vi "SendIntegrationControl.vi"(8 "error in (no error)":errorcluster, 10 "Integration Control Register":T1 items=["UNDEFINED"=0, "NAVX_INTEGRATION_CTL_RESET_VEL_X"=1, "NAVX_INTEGRATION_CTL_RESET_VEL_Y"=2, "NAVX_INTEGRATION_CTL_RESET_VEL_Z"=4, "NAVX_INTEGRATION_CTL_RESET_DISP_X"=8, "NAVX_INTEGRATION_CTL_RESET_DISP_Y"=16, "NAVX_INTEGRATION_CTL_RESET_DISP_Z"=32, "NAVX_INTEGRATION_CTL_RESET_YAW"=128], 11 "navX - I2C in":refnum<class "navX - I2C.lvclass">) -> (0 "error out":errorcluster, 3 "navX - I2C out":refnum<class "navX - I2C.lvclass">)   [LabVIEW 2015, in "navX Library v3.lvlib" / "navX - I2C.lvclass"]
uses:
  navX - I2C.lvclass
  navX - Interface/_TypeDefs/IntegrationControlRegisterTypeDef.ctl
  navX Registry Cache/_TypeDefs/DeviceRegistryTypeDef.ctl
  navX - I2C.lvclass/navX - I2C.ctl
  navX - Interface/navX - Interface.lvclass
  navX Registry Cache/navX Registry Cache.lvclass
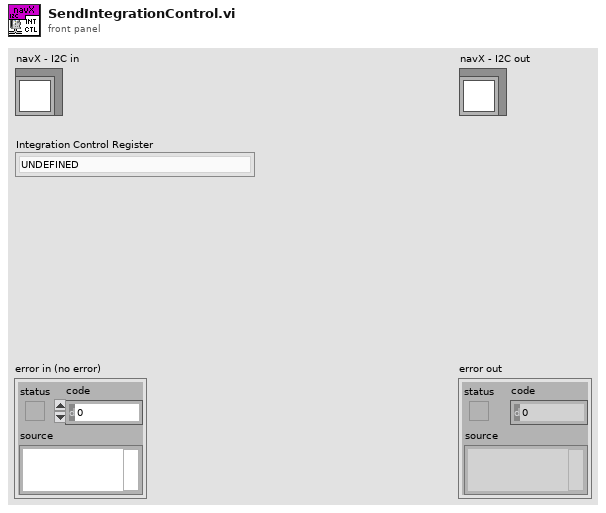
[diagram p1: front panel]
types:
  T1 = typedef "navX Library v3.lvlib/navX - Interface.lvclass/IntegrationControlRegisterTypeDef.ctl" = u8
  T2 = typedef "navX Library v3.lvlib/navX Registry Cache.lvclass/DeviceRegistryTypeDef.ctl" = u8
  T3 = typedef "WPI_I2CDevRef.ctl" = cluster{"DevStatus":errorcluster, "Device Address":u8, "Handle":i32, "I2C Bus":T4}
  T4 = typedef "i2c_bus.ctl" = enum16{"I2C On-Board", "I2C MXP", "Invalid"}
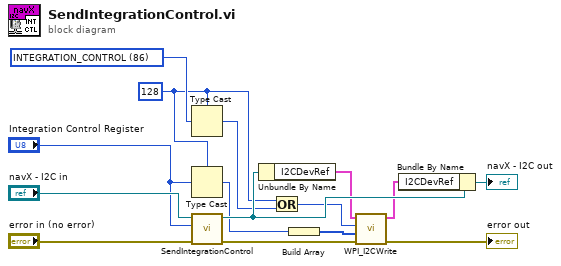
[diagram p0: block diagram]
diagram:
  w4 = u8 128
  w7 = T2 86 items=["WHOAMI"=0, "HW_REV"=1, "FW_VER_MAJOR"=2, "FW_VER_MINOR"=3, "UPDATE_RATE_HZ"=4, "ACCEL_FSR_G"=5, "GYRO_FSR_DPS"=6, "OP_STATUS"=8, "CAL_STATUS"=9, "SELFTEST_STATUS"=10, "CAPABILITY_FLAGS_L"=11, "CAPABILITY_FLAGS_H"=12, "SENSOR_STATUS"=16, "TIMESTAMP"=18, "YAW"=22, "ROLL"=24, "PITCH"=26, "HEADING"=28, "FUSED_HEADING"=30, "ALTITUDE_I"=32, "ALTITUDE_D"=34, "LINERA_ACC_X"=36, "LINERA_ACC_Y"=38, "LINERA_ACC_Z"=40, "QUAT_W"=42, "QUAT_X"=44, "QUAT_Y"=46, "QUAT_Z"=48, "MPU_TEMP_C"=50, "GYRO_X"=52, "GYRO_Y"=54, "GYRO_Z"=56, "ACC_X"=58, "ACC_Y"=60, "ACC_Z"=62, "MAG_X"=64, "MAG_Y"=66, "MAG_Z"=68, "PRESSURE_I"=70, "PRESSURE_D"=72, "PRESSURE_TEMP"=74, "YAW_OFFSET"=76, "QUAT_OFFSET_W"=78, "QUAT_OFFSET_X"=80, "QUAT_OFFSET_Y"=82, "QUAT_OFFSET_Z"=84, "INTEGRATION_CONTROL"=86, "VELOCITY_X"=88, "VELOCITY_Y"=92, "VELOCITY_Z"=96, "DISPLACMENT_X"=100, "DISPLACMENT_Y"=104, "DISPLACEMENT_Z"=108] ("Device Register")
  n1 = Type Cast(type=w4, x=w7) -> (*(type *) &x=w5:u8)
  n2 = Type Cast(type=w4, x="Integration Control Register") -> (*(type *) &x=w2:u8)
  n3 = call-parent "SendIntegrationControl.vi"("error in (no error)"="error in (no error)", "Integration Control Register"="Integration Control Register", "navX - Interface in"="navX - I2C in") -> ("error out"=w9:errorcluster, "navX - Interface out"=w12:refnum<class "navX - I2C.lvclass">)  [unwired: 7 in]
  n4 = Unbundle By Name(w12) -> ("I2CDevRef"=w11:T3)
  n5 = Or(x=w4, y=w5) -> (x .or. y?=w6:u8)
  n6 = Build Array(w2) -> (w1:u8[])
  n7 = call <vilib>:"WPI_I2CWrite.vi"("error in (no error)"=w9, "I2CDataToSend"=w1, "I2CRegister"=w6, "I2CDevRef"=w11) -> ("error out"=→"error out":errorcluster, "I2CDevRef"=w10:T3)  [unwired: 6 in]
  n8 = Bundle By Name(cluster=w12, "I2CDevRef"=w10) -> (→"navX - I2C out":refnum<class "navX - I2C.lvclass">)
